vi "NeoProducer.vi"(7 "queue in":refnum<queue>, 8 "Error In":errorcluster, 10 "NeoParam 2":T1, 11 "Handle":i32) -> (0 "Error Out":errorcluster)   [LabVIEW 2014]
uses:
  <userlib>/AndorSDK3/Data/GetPixelData16.vi
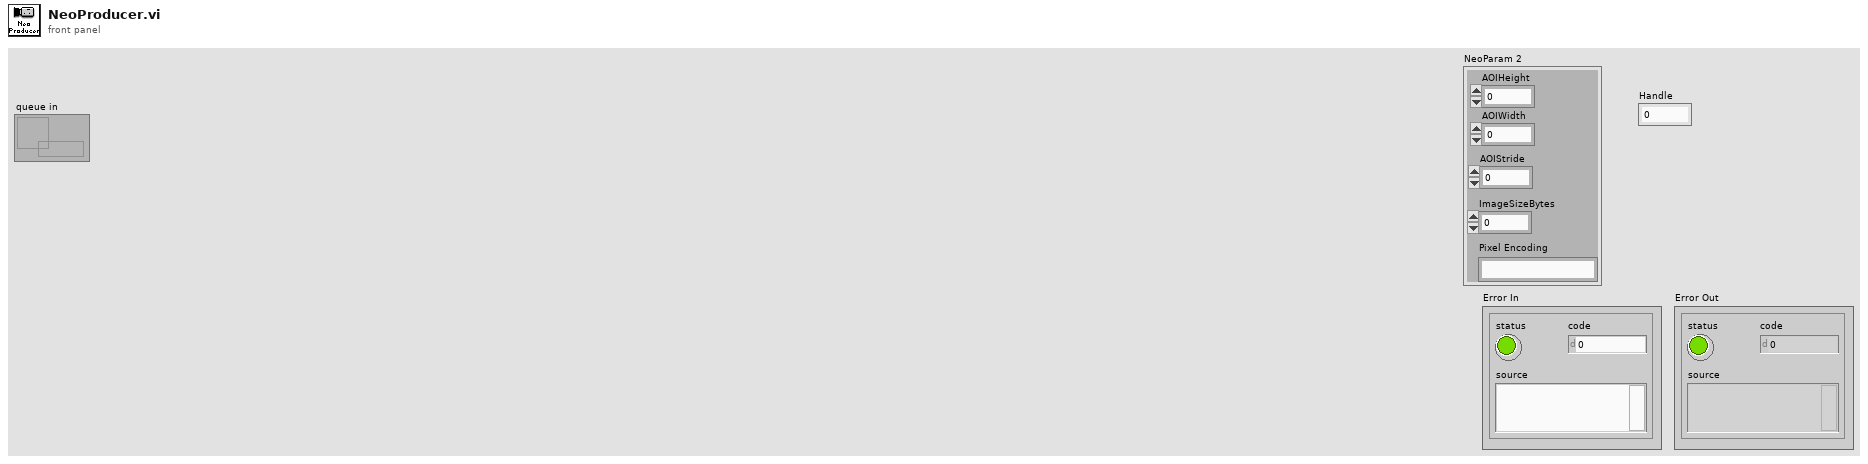
[diagram p1: front panel]
types:
  T1 = cluster{"AOIHeight":i64, "AOIWidth":i64, "AOIStride":i64, "ImageSizeBytes":i64, "Pixel Encoding":string}
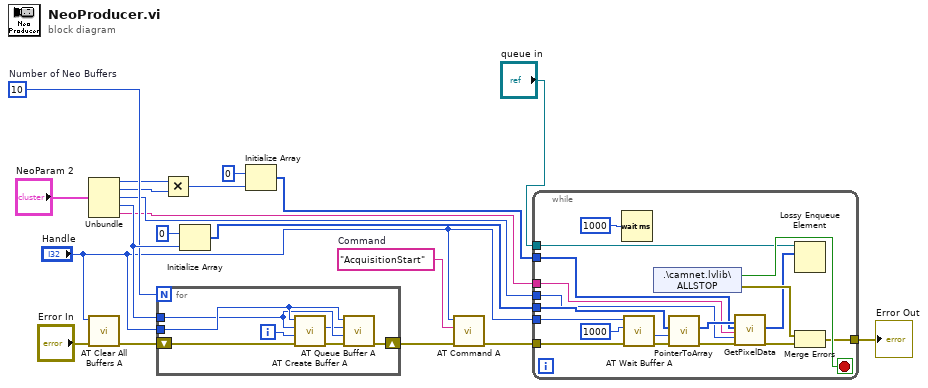
[diagram p0: block diagram]
diagram:
  w14 = "AcquisitionStart"  # Command
  w13 = 10  # Number of Neo Buffers
  n1 = Unbundle("NeoParam 2") -> ("AOIHeight"=w8:i64, "AOIWidth"=w7:i64, "AOIStride"=w4:i64, "ImageSizeBytes"=w17:i64, "Pixel Encoding"=w2:string)
  n2 = call <userlib>:"AT Clear All Buffers A.vi"("error in (no error)"="Error In", "Handle"="Handle") -> ("error out"=w5:errorcluster)  [unwired: 8 in, 1 out]
  n3 = for {
    N: w13 -> [_]
    tunnel: "Handle" -> [w24]
    shift-right: [w25] -> w16
    shift-left: w5 -> [w27]
    tunnel: w17 -> [w22]
    i -> [w23]
    n4 = call <userlib>:"AT Create Buffer A.vi"("error in (no error)"=w27, "Buffer"=w23, "Size"=w22, "Handle"=w24) -> ("error out"=w26:errorcluster, "Buffer out"=w21:u64)  [unwired: 5 in, 1 out]
    n5 = call <userlib>:"AT Queue Buffer A.vi"("error in (no error)"=w26, "PtrSize"=w22, "Ptr"=w21, "Handle"=w24) -> ("error out"=w25:errorcluster)  [unwired: 6 in, 1 out]
  }
  n6 = Multiply(x=w8, y=w7) -> (x*y=w9:i64)
  n7 = Initialize Array(u8 0, w17) -> (w11:u8[])
  n8 = Initialize Array(u16 0, w9) -> (w6:u16[])
  n9 = call <userlib>:"AT Command A.vi"("error in (no error)"=w16, "Feature"=w14, "Handle"="Handle") -> ("error out"=w15:errorcluster)  [unwired: 7 in, 1 out]
  n10 = while {
    tunnel: w15 -> [w39]
    tunnel: [w43] -> w20
    tunnel: "queue in" -> [w41]
    tunnel: "Handle" -> [w38]
    tunnel: w11 -> [w35]
    tunnel: w6 -> [w31]
    tunnel: w4 -> [w29]
    tunnel: w2 -> [w28]
    stop <- w45 stop-if-true
    n11 = Wait (ms)(milliseconds to wait=u32 1000) -> ()  [unwired: 1 out]
    n12 = call <userlib>:"AT Wait Buffer A.vi"("error in (no error)"=w39, "Timeout"=u32 1000, "Handle"=w38) -> ("error out"=w37:errorcluster, "Output buffer"=w36:u64)  [unwired: 5 in, 2 out]
    n13 = shared-variable ".\\camnet.lvlib\\ALLSTOP"() -> (w45:bool, error out=w42:errorcluster)  [unwired: 1 in]
    n14 = call <userlib>:"PointerToArray.vi"("error in (no error)"=w37, "Pointer In"=w36, "Array in"=w35) -> ("error out"=w34:errorcluster, "Array out"=w32:u8[])  [unwired: 7 in]
    n15 = call-poly <userlib>:"GetPixelData.vi"("Input buffer"=w32, "Output buffer in"=w31, "Pixel Encoding"=w28, "Stride"=w29, "error in (no error)"=w34) -> ("Output buffer out"=w30:u16[], "error out"=w33:errorcluster)  [unwired: 12 in, 1 out]
    n16 = Lossy Enqueue Element(queue=w41, element=w30) -> ()  [unwired: 1 in, 4 out]
    n17 = Merge Errors(w42, w33) -> (w43:errorcluster)
  }
  "Error Out" <- w20
